vi "Error Query.vi"(8 "error in (no error)":errorcluster, 11 "VISA resource name":refnum<visa-resource-name>) -> (0 "error out":errorcluster, 1 "Error Message":string, 2 "Error Code":i32[](array[numeric]), 3 "VISA resource name out":refnum<visa-resource-name>)   [LabVIEW 2017, in "ADCMT 6240.lvlib"]
doc: "Queries the instrument for any errors in the instrument's error queue. It will continue to read errors until all errors have been read from the instrument. Any errors will be returned in the <B>error out</B> control.\n\n<B>Note:</B>\nThis VI is called automatically by most driver VIs so it is not usually necessary to call this in an application."
uses:
  ADCMT 6240.lvlib
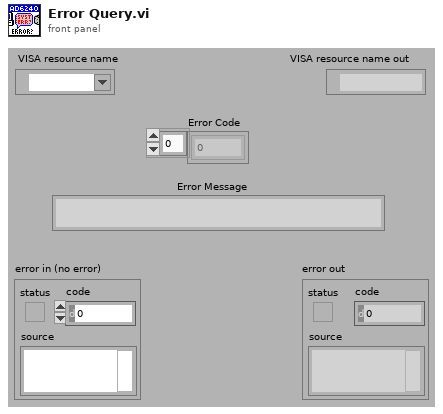
[diagram p1: front panel]
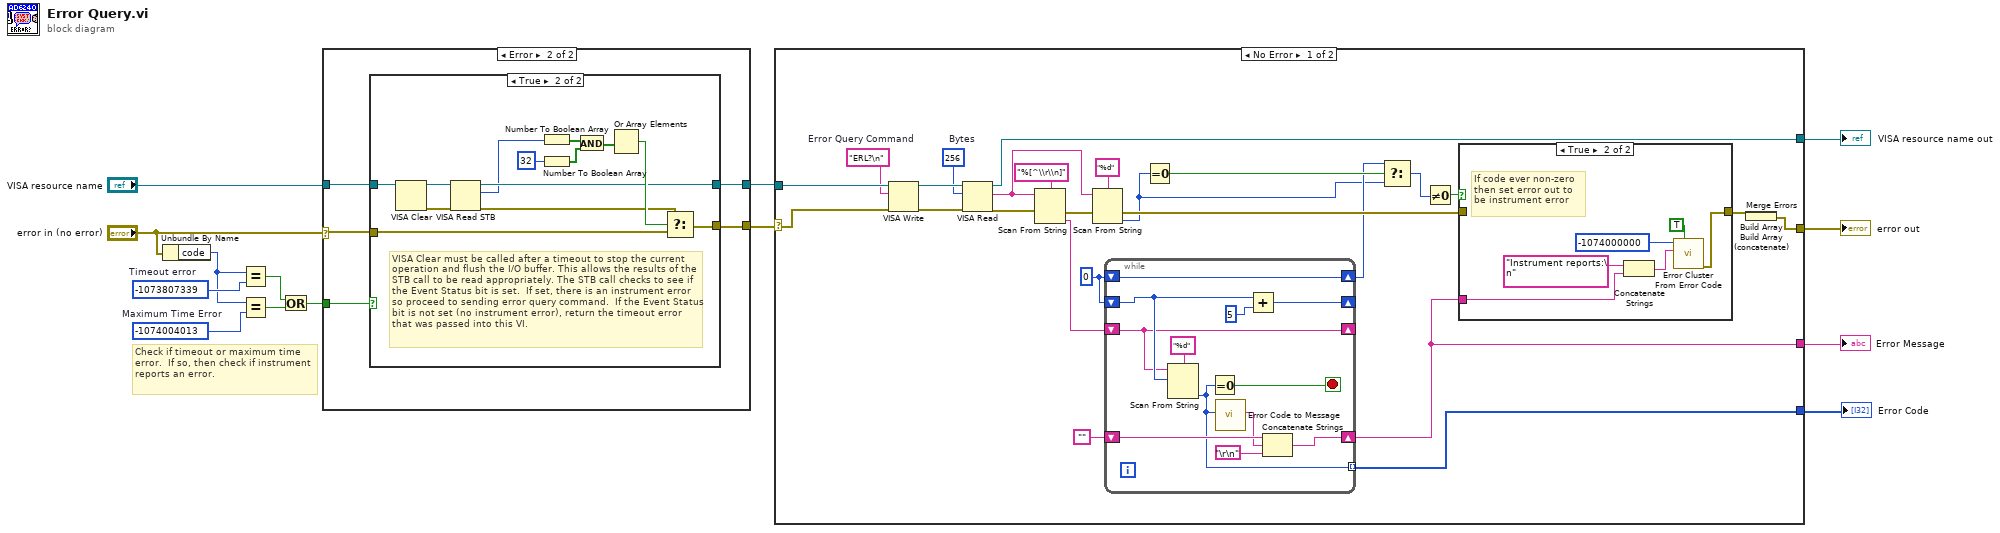
[diagram p0: block diagram]
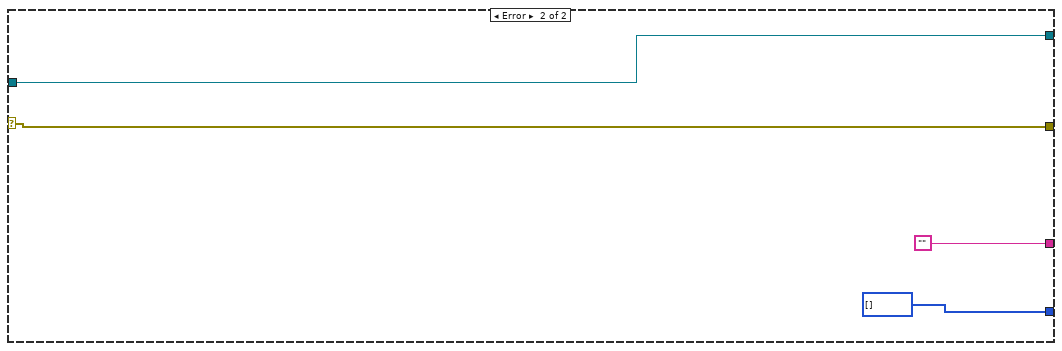
[diagram p5: hidden frame]
diagram:
  w5 = -1074004013  # Maximum Time Error
  w7 = -1073807339  # Timeout error
  # "Check if timeout or maximum time error.  If so, then check if instrument reports an error."
  n1 = Unbundle By Name("error in (no error)") -> ("code"=w6:i32)
  n2 = Equal?(x=w6, y=w7) -> (x = y?=w3:bool)
  n3 = Equal? ("等しい?")(x=w6, y=w5) -> (x = y?=w4:bool)
  n4 = Or(x=w3, y=w4) -> (x .or. y?=w2:bool)
  n5 = case "ケースストラクチャ" shown="Error" "error in (no error)" {
    selector: "error in (no error)" -> [w15 w19]
    tunnel: "VISA resource name" -> [w16 w21]
    tunnel: [w16 w20] -> w9
    tunnel: [w15 w18] -> w10
    tunnel: w2 -> [_ w17]
    frame No Error {
    }
    frame Error {
      n6 = case "ケースストラクチャ" shown="True" w17 {
        tunnel: w21 -> [w23 w29]
        tunnel: [w23 w26] -> w20
        tunnel: w19 -> [w22 w32]
        tunnel: [w22 w31] -> w18
        frame False {
          # "Error code not a timeout, so best to pass on to user."
        }
        frame True {
          # "VISA Clear must be called after a timeout to stop the current operation and flush the I/O buffer. This allows the results of the  STB call to be read appropriately. The STB call checks to see if the Event Status bit is set.  If set, there is an instrument error so proceed to sending error query command.  If the Event Status bit is not set (no instrument error), return the timeout error that was passed into this VI."
          n7 = VISA Clear ("VISAクリア")(VISA resource name=w29) -> (VISA resource name out=w28:refnum<visa-resource-name>, error out=w27:errorcluster)  [unwired: 1 in]
          n8 = VISA Read STB ("VISA STB読み取り")(8:w27, 11:w28) -> (0:w25:errorcluster, 2:w24:u16, 3:w26:refnum<visa-resource-name>)
          n9 = Number To Boolean Array ("数値をブール配列に変換")(number=w24) -> (Boolean array=w33:bool[])
          n10 = Number To Boolean Array ("数値をブール配列に変換")(number=32) -> (Boolean array=w35:bool[])
          n11 = And(x=w33, y=w35) -> (x .and. y?=w34:bool[])
          n12 = Or Array Elements ("配列要素のOr")(Boolean array=w34) -> (logical OR=w30:bool)
          n13 = Select ("選択")(t=w25, s=w30, f=w32) -> (s? t:f=w31:errorcluster)
        }
      }
    }
  }
  n14 = case "ケースストラクチャ" shown="No Error" w10 {
    selector: w10 -> [w56 w83]
    tunnel: [w63 w86] -> w14
    tunnel: w9 -> [w62 w86]
    tunnel: [w61 w83] -> w13
    tunnel: [w44 "" ("空文字列定数")] -> w12
    tunnel: [w43 i32[] []] -> w11
    frame No Error {
      w40 = 0
      w54 = u32 256  # Bytes
      w52 = "ERL?\n"  # Error Query Command
      n15 = VISA Write ("VISA書き込み")(VISA resource name=w62, write buffer=w52, error in (no error)=w56) -> (VISA resource name out=w55:refnum<visa-resource-name>, error out=w53:errorcluster)  [unwired: 1 out]
      n16 = VISA Read ("VISA読み取り")(VISA resource name=w55, byte count=w54, error in (no error)=w53) -> (VISA resource name out=w63:refnum<visa-resource-name>, read buffer=w49:string, error out=w48:errorcluster)  [unwired: 1 out]
      n17 = Scan From String ("文字列からスキャン")(format string="%[^\\r\\n]", input string=w49, error in=w48) -> (error out=w47:errorcluster, output 1=w42:string)  [unwired: 2 in, 2 out]
      n18 = Scan From String ("文字列からスキャン")(format string="%d", input string=w49, error in=w47) -> (error out=w57:errorcluster, output 1=w39:i32)  [unwired: 2 in, 2 out]
      n19 = while "Whileループ" {
        shift-right: [w69] -> w41
        shift-left: w40 -> [w69]
        shift-right: [w71] -> w44
        shift-left: "" ("空文字列定数") -> [w73]
        tunnel: [w68] -> w43 mode=indexing
        shift-right: [w64] -> _
        shift-left: w42 -> [w64]
        shift-right: [w66] -> _
        shift-left: w40 -> [w65]
        stop <- w70 stop-if-true
        n20 = Scan From String ("文字列からスキャン")(format string="%d", input string=w64, initial scan location=w65) -> (output 1=w68:i32)  [unwired: 2 in, 3 out]
        n21 = Equal To 0? ("0に等しい?")(x=w68) -> (x = 0?=w70:bool)
        n22 = call "Error Code to Message.vi"("Error Code (0)"=w68) -> ("Error Message"=w72:string)  [unwired: 10 in]
        n23 = Add ("和")(x=w65, y=5) -> (x+y=w66:i32)
        n24 = Concatenate Strings ("文字列連結")(w73, w72, "\r\n" ("復帰改行定数")) -> (w71:string)
      }
      n25 = Equal To 0? ("0に等しい?")(x=w39) -> (x = 0?=w46:bool)
      n26 = Select ("選択")(t=w41, s=w46, f=w39) -> (s? t:f=w58:i32)
      n27 = Not Equal To 0? ("0に等しくない?")(x=w58) -> (x != 0?=w60:bool)
      n28 = case "ケースストラクチャ" shown="True" w60 {
        tunnel: w44 -> [_ w81]
        tunnel: [w76 w77] -> w59
        tunnel: w57 -> [w76 _]
        frame False {
        }
        frame True {
          # "If code ever non-zero\nthen set error out to\nbe instrument error"
          n29 = Concatenate Strings ("文字列連結")("Instrument reports:\n" ("Source"), w81) -> (w78:string)
          n30 = call <vilib>:"Error Cluster From Error Code.vi"("show call chain? (False)"=TRUE, "error message (\"\")"=w78, "error code (0)"=-1074000000 ("Code")) -> ("error out"=w77:errorcluster)  [unwired: 6 in]
        }
      }
      n31 = Build Array(w59) -> (w38:errorcluster[])
      n32 = Build Array (concatenate)(w38) -> (w37:errorcluster[])
      n33 = Merge Errors(w37) -> (w61:errorcluster)
    }
    frame Error {
    }
  }
  "VISA resource name out" <- w14
  "error out" <- w13
  "Error Message" <- w12
  "Error Code" <- w11
